vi "Set Internal Max.vi"(6 "parseError? T:Yes":bool=TRUE, 8 "error in (no error)":errorcluster, 10 "InternMax (50.00 °C)":dbl=50.0, 11 "VISA resource name":refnum<visa-resource-name>) -> (0 "error out":errorcluster, 3 "VISA resource name out":refnum<visa-resource-name>)   [LabVIEW 2015, in "JULABO DeviceDriver.lvlib"]
doc: "This VI adjusts the upper temperature limit for the internal temperature during external temperature control. <B>InternMax</B> and <B>InternMin</B> (see JULABO_Configure_SetInternMin.vi) determine fixed limits for the temperature within the internal bath. The temperature controller cannot exceed these limits even if it would be necessary for achieving the temperature in an external system. Therefore it is possible that the external setpoint cannot be achieved."
uses:
  JULABO DeviceDriver.lvlib
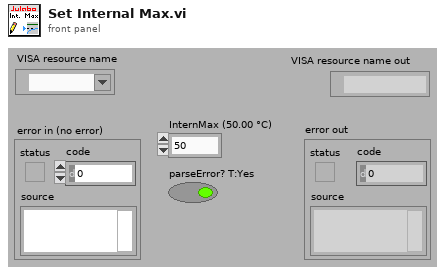
[diagram p1: front panel]
types:
  T1 = typedef "JULABO DeviceDriver.lvlib/InstrumentType.ctl" = enum8{"Default", "FC-Series", "HT30/HT60", "LC4"}
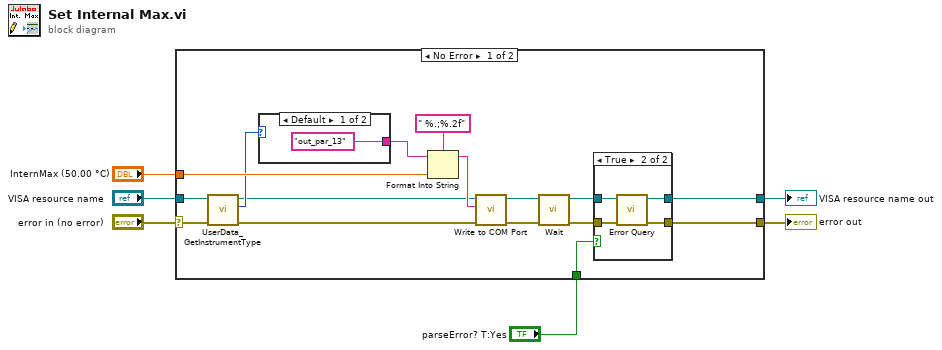
[diagram p0: block diagram]
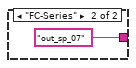
[diagram p2: hidden frame]
diagram:
  n1 = case shown="No Error" "error in (no error)" {
    selector: "error in (no error)" -> [w10 w31]
    tunnel: "VISA resource name" -> [w11 w32]
    tunnel: [w21 w31] -> w5
    tunnel: [w20 w32] -> w4
    tunnel: "InternMax (50.00 °C)" -> [w22 _]
    tunnel: "parseError? T:Yes" -> [w19 _]
    frame No Error {
      n2 = call "UserData_GetInstrumentType.vi"("Fehler (Eingang)"=w10, "VISA resource name in"=w11) -> ("Fehler (Ausgang)"=w9:errorcluster, "InstrumentType"=w12:T1, "VISA resource name out"=w8:refnum<visa-resource-name>)  [unwired: 3 in]
      n3 = case shown="Default" w12 {
        tunnel: ["out_par_13" "out_sp_07"] -> w7
        frame Default {
        }
        frame "FC-Series" {
        }
      }
      n4 = Format Into String(format string=" %.;%.2f", initial string=w7, w22) -> (resulting string=w13:string)  [unwired: 1 in, 1 out]
      n5 = call "Write to COM Port.vi"("error in"=w9, "Command (input)"=w13, "VISA resource name in"=w8) -> ("error out"=w17:errorcluster, "VISA resource name out"=w18:refnum<visa-resource-name>)  [unwired: 7 in]
      n6 = call "Wait.vi"("error in"=w17, "VISA resource name in"=w18) -> ("error out"=w15:errorcluster, "VISA resource name out"=w16:refnum<visa-resource-name>)  [unwired: 4 in]
      n7 = case shown="True" w19 {
        tunnel: w16 -> [w26 w30]
        tunnel: w15 -> [w25 w29]
        tunnel: [w26 w28] -> w20
        tunnel: [w25 w27] -> w21
        frame False {
        }
        frame True {
          n8 = call "Error Query.vi"("error in (no error)"=w29, "VISA resource name"=w30) -> ("error out"=w27:errorcluster, "VISA resource name out"=w28:refnum<visa-resource-name>)  [unwired: 6 in, 2 out]
        }
      }
    }
    frame Error {
    }
  }
  "error out" <- w5
  "VISA resource name out" <- w4
